vi "Set DO State (manual mode).vi"(8 "error in (no error)":errorcluster, 9 "State":bool, 10 "DO IOName":string, 11 "DAQ":refnum<class "DAQ.lvclass">) -> (0 "error out":errorcluster, 3 "DAQ":refnum<class "DAQ.lvclass">)   [LabVIEW 2017, in "DAQ.lvclass"]
doc: "Developed by Kevin Thompson\nkevin@thompsonengineering.net\n\nCopyright 2018-2020\nThompson Engineering, LLC\nCall this Set DO State method for setting digital output states in manually operated test panel UI's."
uses:
  DAQ.lvclass
  DataTypes/TD DAQ Output EventSenderMode-enum.ctl
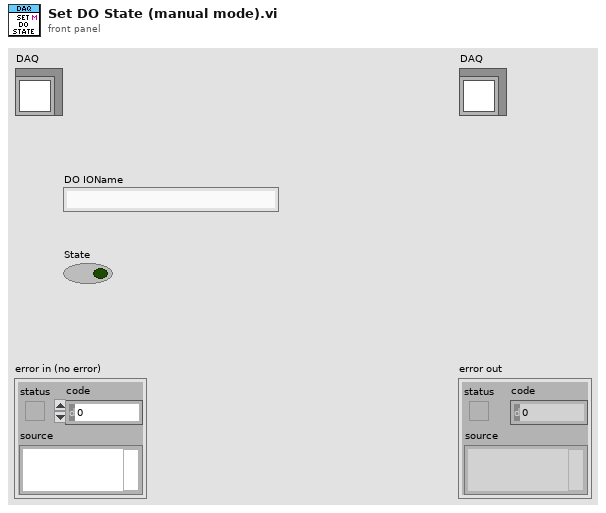
[diagram p1: front panel]
types:
  T1 = typedef "DAQ.lvclass/TD DAQ Output EventSenderMode-enum.ctl" = enum16{"manual", "automation"}
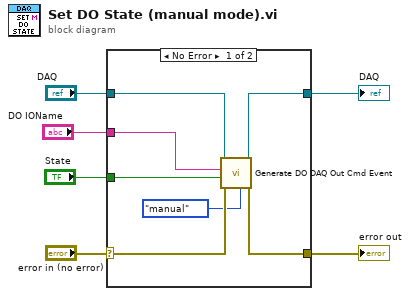
[diagram p0: block diagram]
diagram:
  n1 = case shown="No Error" "error in (no error)" {
    selector: "error in (no error)" -> [w13 w15]
    tunnel: [w12 w15] -> w5
    tunnel: [w10 w14] -> w3
    tunnel: "DAQ" -> [w11 w14]
    tunnel: "DO IOName" -> [w7 _]
    tunnel: "State" -> [w8 _]
    frame No Error {
      n2 = call "Generate DO DAQ Out Cmd Event.vi"("mode (manual)"=TD_DAQ_Output_EventSenderMode-enum."manual" ("mode (automation)"), "error in (no error)"=w13, "BoolState"=w8, "DO IOName"=w7, "DAQ"=w11) -> ("error out"=w12:errorcluster, "DAQ"=w10:refnum<class "DAQ.lvclass">)  [unwired: 5 in]
    }
    frame Error {
    }
  }
  "error out" <- w5
  "DAQ" <- w3
